vi "MT Format Constellation.vi"(0 "waveform":T2={"t0"=0.0, "dt"=1.0, "Y"=[]} {"Y" format="%.3f"; "dt" format="%^.2e"; "t0" format="%.4f"}, 1 "constellation reference":refnum<vi>, 5 "samples per symbol":i32=16, 7 "autoscale":bool, 11 "error in (no error)":errorcluster) -> (4 "constellation graph":T1(array[cluster]) {"oversampled data" format="%.2f"; "constellation" format="%.2f"}, 15 "error out":errorcluster)   [LabVIEW 2020, in "niDMT.lvlib"]
doc: "Prepares a signal for presentation on a graph that shows the detected symbol locations and the transitions between those symbols. The VI specifies a complex-valued waveform and displays a constellation plot of the waveform contents."
uses:
  <vilib>/addons/Modulation/niDMT.lvlib
  <vilib>/addons/Modulation/Analog/controls/Complex Data Waveform.ctl
  <vilib>/addons/Modulation/niAMT.lvlib
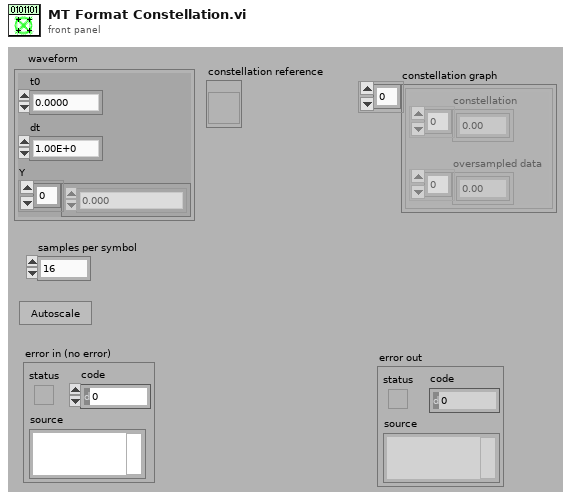
[diagram p1: front panel]
types:
  T1 = cluster{"constellation":dbl[], "oversampled data":dbl[]}[]
  T2 = typedef "niAMT.lvlib/Complex Data Waveform.ctl" = cluster{"t0":dbl, "dt":dbl, "Y":cdb[]}
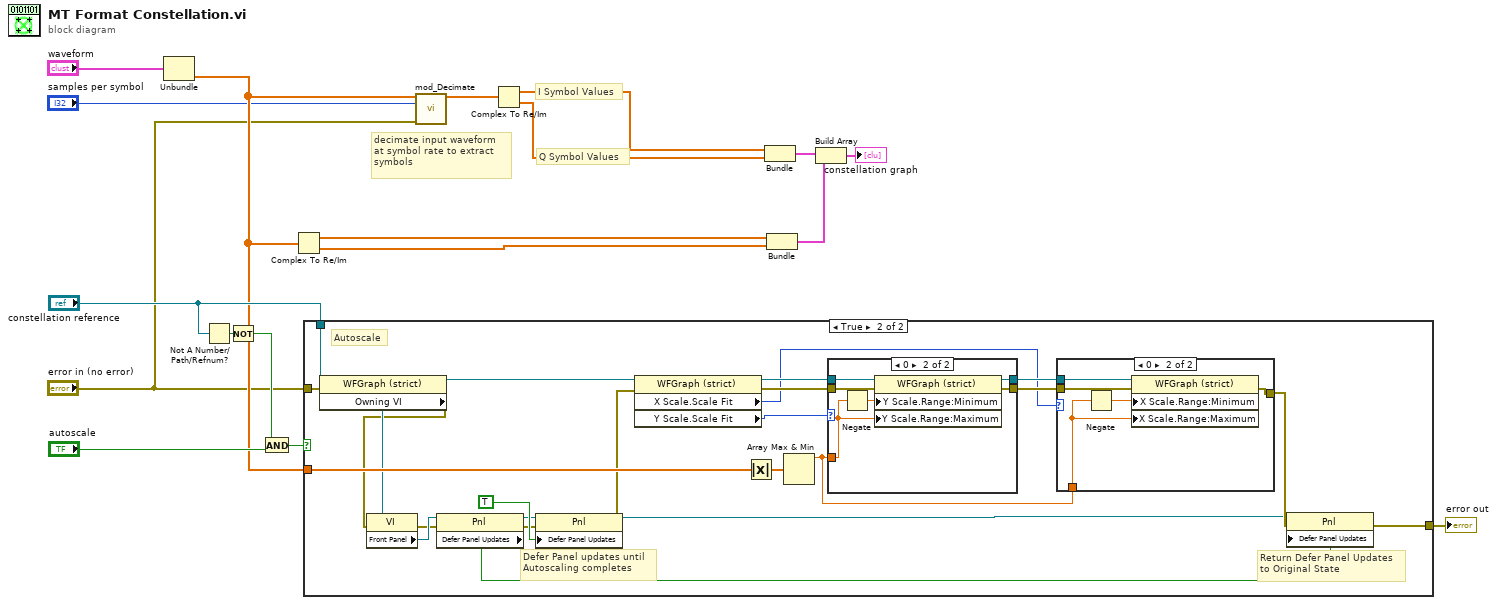
[diagram p0: block diagram]
diagram:
  # "Q Symbol Values"
  # "I Symbol Values"
  # "decimate input waveform\nat symbol rate to extract\nsymbols"
  n1 = Unbundle("waveform") -> ("Y"=w5:cdb[])  [unwired: 2 out]
  n2 = Not A Number/Path/Refnum?(number/path/refnum="constellation reference") -> (NaN/Path/Refnum?=w17:bool)
  n3 = Not(x=w17) -> (.not. x?=w15:bool)
  n4 = And(x=w15, y="autoscale") -> (x .and. y?=w18:bool)
  n5 = Complex To Re/Im(x + iy=w5) -> (x=w14:dbl[], y=w13:dbl[])
  n6 = case shown="True" w18 {
    tunnel: w5 -> [_ w41]
    tunnel: "constellation reference" -> [_ w32]
    tunnel: [w19 w25] -> w11
    tunnel: "error in (no error)" -> [w19 w33]
    frame False {
    }
    frame True {
      # "Defer Panel updates until\nAutoscaling completes"
      # "Autoscale"
      # "Return Defer Panel Updates\nto Original State"
      n7 = property class="WFGraph (strict)"(reference=w32, error in=w33) -> (reference out=w34:refnum<vi>, error out=w30:errorcluster, "Owning VI"=w31:refnum<vi>)
      n8 = property class="VI"(reference=w31, error in=w30) -> (error out=w21:errorcluster, "Front Panel"=w24:refnum<vi>)  [unwired: 1 out]
      n9 = property class="Pnl"(reference=w24, error in=w21) -> (reference out=w23:refnum<vi>, error out=w22:errorcluster, "Defer Panel Updates"=w20:bool)
      n10 = property class="Pnl"(reference=w23, error in=w22, "Defer Panel Updates"=TRUE) -> (reference out=w26:refnum<vi>, error out=w28:errorcluster)
      n11 = property class="WFGraph (strict)"(reference=w34, error in=w28) -> (reference out=w36:refnum<vi>, error out=w37:errorcluster, "X Scale.Scale Fit"=w35:u8, "Y Scale.Scale Fit"=w43:u8)
      n12 = Absolute Value(x=w41) -> (abs(x)=w42:dbl[])
      n13 = Array Max & Min(array=w42) -> (max value=w40:dbl)  [unwired: 3 out]
      n14 = case shown="0" w43 {
        tunnel: [w51 w56] -> w39
        tunnel: w40 -> [_ w55]
        tunnel: [w50 w54] -> w38
        tunnel: w37 -> [w51 w52]
        tunnel: w36 -> [w50 w53]
        frame 1, Default {
        }
        frame 0 {
          n15 = Negate(x=w55) -> (-x=w57:dbl)
          n16 = property class="WFGraph (strict)"(reference=w53, error in=w52, "Y Scale.Range:Minimum"=w57, "Y Scale.Range:Maximum"=w55) -> (reference out=w54:refnum<vi>, error out=w56:errorcluster)
        }
      }
      n17 = case shown="0" w35 {
        tunnel: [w44 w49] -> w27
        tunnel: w39 -> [w44 w46]
        tunnel: w40 -> [_ w47]
        tunnel: w38 -> [_ w45]
        frame 1, Default {
        }
        frame 0 {
          n18 = Negate(x=w47) -> (-x=w48:dbl)
          n19 = property class="WFGraph (strict)"(reference=w45, error in=w46, "X Scale.Range:Minimum"=w48, "X Scale.Range:Maximum"=w47) -> (error out=w49:errorcluster)  [unwired: 1 out]
        }
      }
      n20 = property class="Pnl"(reference=w26, error in=w27, "Defer Panel Updates"=w20) -> (error out=w25:errorcluster)  [unwired: 1 out]
    }
  }
  "error out" <- w11
  n21 = call <vilib>:"mod_Decimate.vi"("Signal In"=w5, "Samples Per Symbol (16)"="samples per symbol", "error in (no error)"="error in (no error)") -> ("Signal Out"=w4:cdb[])  [unwired: 1 in, 11 out]
  n22 = Complex To Re/Im(x + iy=w4) -> (x=w7:dbl[], y=w6:dbl[])
  n23 = Bundle(w7, w6) -> (w2:cluster{dbl[], dbl[]})  [unwired: 1 out]
  n24 = Bundle(w14, w13) -> (w12:cluster{dbl[], dbl[]})  [unwired: 1 out]
  n25 = Build Array(w2, w12) -> (→"constellation graph":cluster{dbl[], dbl[]}[])
